vi "Test Handle LogRecord.vi"(8 "error in (no error)":errorcluster) -> (0 "error out":errorcluster)   [LabVIEW 2016, in "UT_UserEventHandler.lvlib"]
doc: "Test the processing of an LogRecord."
uses:
  UT_UserEventHandler.lvlib
  Source/HSE-Logger/LogLevel.ctl
  Source/HSE-Logger/LogRecord/LogRecord.lvclass/LogRecord.ctl
  <vilib>/addons/_JKI Toolkits/Caraya/classes/Assert/Assert Equal Value and Type_Variant.vi
  <vilib>/addons/_JKI Toolkits/Caraya/classes/Assert/Assert Error.vi
  Source/HSE-Logger/Handler/UserEventHandler/UserEventHandler.lvclass
  <vilib>/addons/_JKI Toolkits/Caraya/classes/Test/Test.lvclass
  Source/HSE-Logger/hse-logger.lvlib
  Source/HSE-Logger/LogRecord/LogRecord.lvclass
  <vilib>/addons/_JKI Toolkits/Caraya/classes/Assert/Assert.lvclass
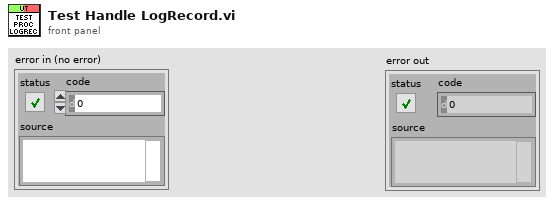
[diagram p1: front panel]
types:
  T1 = typedef "hse-logger.lvlib/LogLevel.ctl" = enum16{"DEBUG", "INFO", "WARNING", "ERROR", "CRITICAL"}
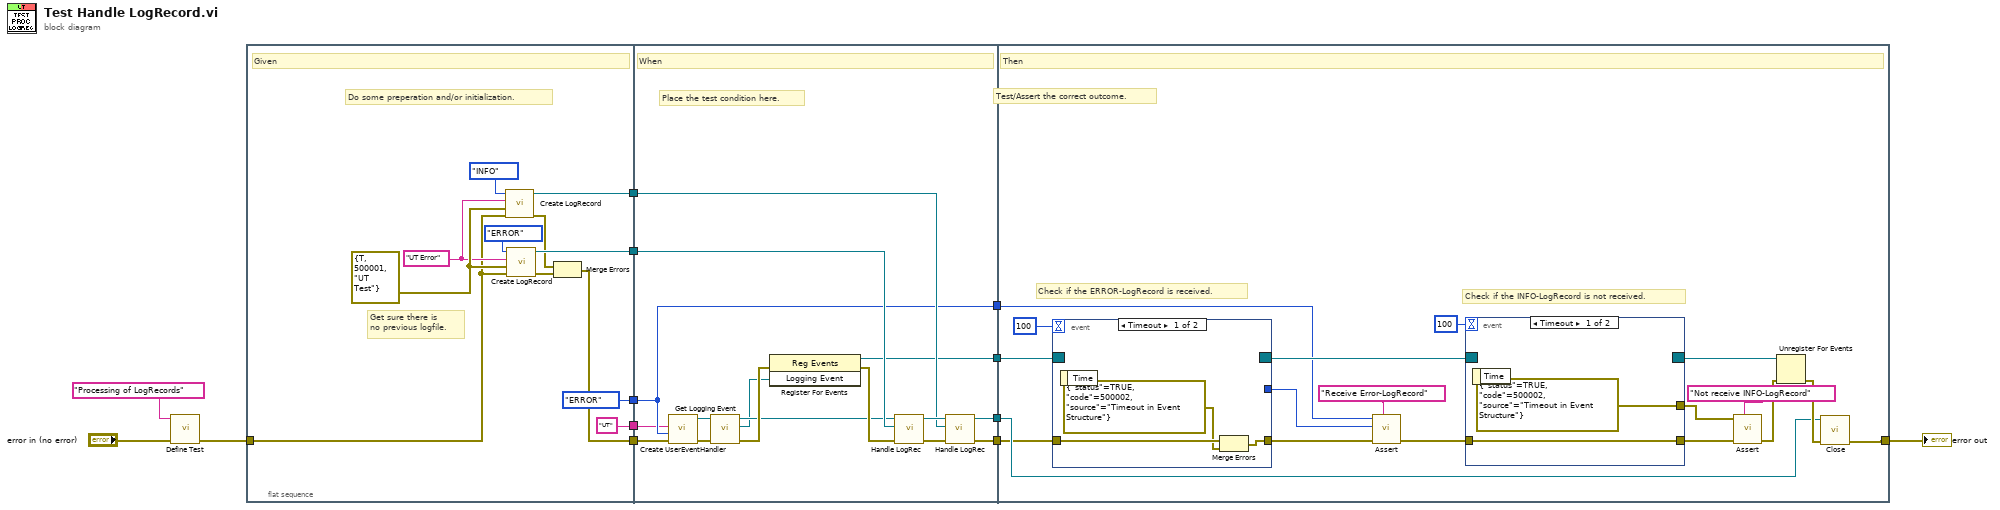
[diagram p0: block diagram]
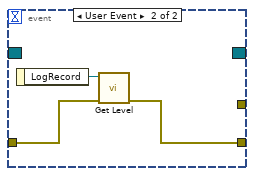
[diagram p2: hidden frame]
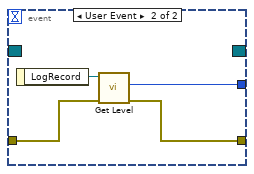
[diagram p3: hidden frame]
diagram:
  n1 = call <vilib>:"Define Test.vi"("error in (no error)"="error in (no error)", "Label (VI Title)"="Processing of LogRecords") -> ("error out"=w10:errorcluster)  [unwired: 8 in, 1 out]
  n2 = flat-sequence {
    tunnel: w10 -> [w14]
    tunnel: [w17] -> w13
    tunnel: [LogLevel."ERROR" ("Level")] -> w8
    tunnel: ["UT" ("Name")] -> w7
    tunnel: [w22] -> w5
    tunnel: [w15] -> w4
    tunnel: w13 -> [w35]
    tunnel: w8 -> [w27]
    tunnel: w7 -> [w26]
    tunnel: [w27] -> w6
    tunnel: w5 -> [w39]
    tunnel: w4 -> [w36]
    tunnel: [w34] -> w3
    tunnel: [w33] -> w2
    tunnel: [w28] -> w1
    tunnel: [w53] -> w12
    tunnel: w6 -> [w48]
    tunnel: w3 -> [w51]
    tunnel: w2 -> [w54]
    tunnel: w1 -> [w52]
    frame #0 {
      w19 = errorcluster {"status"=TRUE, "code"=500001, "source"="UT Test"} ("Error to Log")
      w18 = "UT Error" ("Message")
      # "Get sure there is\nno previous logfile."
      # "Do some preperation and/or initialization."
      # "Given"
      n3 = call "Create LogRecord.vi"("error in"=w14, "Error to Log"=w19, "Message"=w18, "Level"=LogLevel."INFO") -> ("error out"=w16:errorcluster, "LogRecord out"=w15:refnum<class "LogRecord.lvclass">)  [unwired: 6 in]
      n4 = call "Create LogRecord.vi"("error in"=w14, "Error to Log"=w19, "Message"=w18, "Level"=LogLevel."ERROR") -> ("error out"=w21:errorcluster, "LogRecord out"=w22:refnum<class "LogRecord.lvclass">)  [unwired: 6 in]
      n5 = Merge Errors(w16, w21) -> (w17:errorcluster)
    }
    frame #1 {
      # "Place the test condition here."
      # "When"
      n6 = call "Create UserEventHandler.vi"("error in"=w35, "Level"=w27, "Name"=w26) -> ("error out"=w32:errorcluster, "UserEventHandler out"=w31:refnum<class "UserEventHandler.lvclass">)  [unwired: 7 in]
      n7 = call-dynamic "Get Logging Event.vi"("error in"=w32, "UserEventHandler in"=w31) -> ("error out"=w40:errorcluster, "Logging Event"=w29:refnum<user-event>, "UserEventHandler out"=w30:refnum<class "UserEventHandler.lvclass">)  [unwired: 7 in]
      n8 = register-events(error in=w40, w29) -> (reference out=w28:refnum<event-registration>, error out=w41:errorcluster)  [unwired: 1 in]
      n9 = call-dynamic "Handle LogRec.vi"("error in"=w41, "LogRecord"=w39, "UserEventHandler in"=w30) -> ("error out"=w38:errorcluster, "UserEventHandler out"=w37:refnum<class "UserEventHandler.lvclass">)  [unwired: 7 in]
      n10 = call-dynamic "Handle LogRec.vi"("error in"=w38, "LogRecord"=w36, "UserEventHandler in"=w37) -> ("error out"=w34:errorcluster, "UserEventHandler out"=w33:refnum<class "UserEventHandler.lvclass">)  [unwired: 7 in]
    }
    frame #2 {
      # "Check if the INFO-LogRecord is not received."
      # "Check if the ERROR-LogRecord is received."
      # "Test/Assert the correct outcome."
      # "Then"
      n11 = event shown="[0] Timeout" {
        selector: w52 -> [_ _]
        dyn-events: [_ _] -> w58
        timeout: 100 -> [_ _]
        tunnel: w51 -> [w67 w70]
        tunnel: [w65 w69] -> w50
        tunnel: [_ w68] -> w47
        event Timeout {
          n12 = event-data() -> ()  [unwired: 1 in, 1 out]
          n13 = Merge Errors(w67, errorcluster {"status"=TRUE, "code"=500002, "source"="Timeout in Event Structure"} ("error out")) -> (w65:errorcluster)
        }
        event User Event {
          n14 = event-data() -> ("LogRecord"=w71:refnum<class "LogRecord.lvclass">)  [unwired: 1 in]
          n15 = call "Get Level.vi"("error in"=w70, "LogRecord in"=w71) -> ("error out"=w69:errorcluster, "Level"=w68:T1)  [unwired: 7 in, 1 out]
        }
      }
      n16 = call-poly <vilib>:"Assert.vi"("Label"="Receive Error-LogRecord", "error in (no error)"=w50, "Y"=w47, "X"=w48) -> ("error out"=w49:errorcluster)  [unwired: 6 in, 1 out]
      n17 = event shown="[0] Timeout" {
        selector: w58 -> [_ _]
        dyn-events: [_ _] -> w56
        timeout: 100 -> [_ _]
        tunnel: w49 -> [w61 w63]
        tunnel: [w61 w62] -> w45
        tunnel: [errorcluster {"status"=TRUE, "code"=500002, "source"="Timeout in Event Structure"} ("error out") _] -> w43
        event Timeout {
          n18 = event-data() -> ()  [unwired: 1 in, 1 out]
        }
        event User Event {
          n19 = event-data() -> ("LogRecord"=w64:refnum<class "LogRecord.lvclass">)  [unwired: 1 in]
          n20 = call "Get Level.vi"("error in"=w63, "LogRecord in"=w64) -> ("error out"=w62:errorcluster)  [unwired: 7 in, 2 out]
        }
      }
      n21 = call-poly <vilib>:"Assert.vi"("Label"="Not receive INFO-LogRecord", "error in (no error)"=w45, "Error?"=w43) -> ("error out"=w44:errorcluster)  [unwired: 7 in, 1 out]
      n22 = Unregister For Events(event registration refnum=w56, error in=w44) -> (error out=w55:errorcluster)
      n23 = call-dynamic "Close.vi"("error in"=w55, "UserEventHandler in"=w54) -> ("error out"=w53:errorcluster)  [unwired: 8 in, 1 out]
    }
  }
  "error out" <- w12
